vi "String SW.vi"(11 "Data In":string) -> (3 "Data Out":string)   [LabVIEW 2016]
uses:
  Core/Assert API Components/Failure Actions.ctl
  Core/Assert API Components/VI References.ctl
  Core/Assert API Components/Assert API Components.lvlib
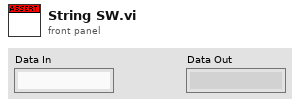
[diagram p1: front panel]
types:
  T1 = typedef "Assert API Components.lvlib/VI References.ctl" = cluster{"Calling VI Ref":refnum<vi>, "Assert VI Ref":refnum<vi>}
  T2 = typedef "Assert API Components.lvlib/Failure Actions.ctl" = enum16{"None", "Log To File", "Pause Execution", "Abort Execution"}
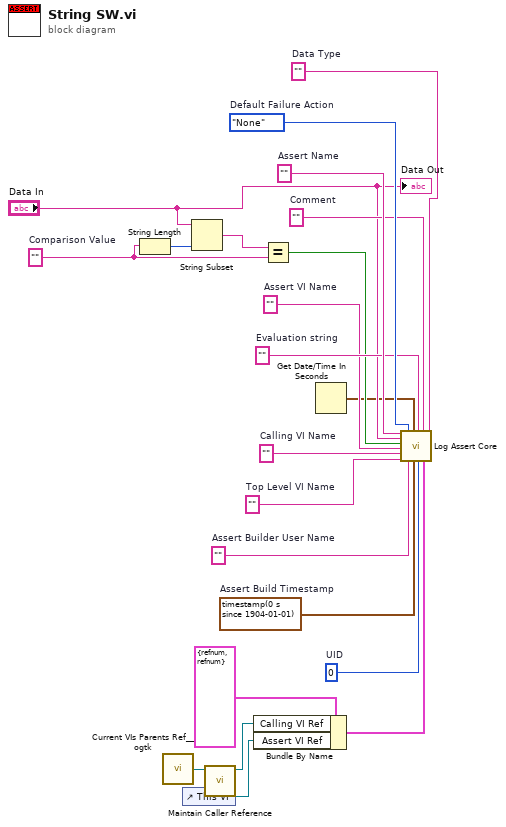
[diagram p0: block diagram]
diagram:
  w2 = ""  # Top Level VI Name
  w4 = 0  # UID
  w5 = ""  # Assert VI Name
  w6 = ""  # Calling VI Name
  w7 = ""  # Assert Builder User Name
  w8 = timestamp(0 s since 1904-01-01)  # Assert Build Timestamp
  w9 = ""  # Data Type
  w20 = ""  # Comment
  w19 = ""  # Evaluation string
  w21 = Failure_Actions."None"  # Default Failure Action
  w22 = ""  # Assert Name
  w15 = ""  # Comparison Value
  n1 = String Length(string=w15) -> (length=w17:i32)
  n2 = call <userlib>:"Current VIs Parents Ref__ogtk.vi"() -> ("Calling VI's Reference"=w12:refnum<vi>)  [unwired: 2 in]
  n3 = control-ref of="This VI"() -> (w11:refnum<vi>)
  n4 = String Subset(string="Data In", length (rest)=w17) -> (substring=w16:string)  [unwired: 1 in]
  n5 = call "Maintain Caller Reference.vi"("VI in"=w12) -> ("VI out"=w1:refnum<vi>)  [unwired: 10 in]
  n6 = Bundle By Name(cluster=T1 {"Calling VI Ref"=refnum, "Assert VI Ref"=refnum} ("VI References"), "Calling VI Ref"=w1, "Assert VI Ref"=w11) -> (w10:T1)
  n7 = Equal?(x=w16, y=w15) -> (x = y?=w14:bool)
  n8 = Get Date/Time In Seconds() -> (seconds since 1Jan1904=w3:timestamp)
  n9 = call "Log Assert Core.vi"("Assert Name"=w22, "Data Value"="Data In", "Status"=w14, "Assert VI Name"=w5, "Calling VI Name"=w6, "Top Level VI Name"=w2, "Failure Action"=w21, "Assert Builder User Name"=w7, "Last Update"=w3, "Assert Build Timestamp"=w8, "Evaluation String"=w19, "Assert VI UID"=w4, "Comment"=w20, "VI References"=w10, "Data Type"=w9) -> ()  [unwired: 5 in]
  "Data Out" <- "Data In"
